vi "WriteAndClosePatientDateInfoFile.vi"(8 "error in (no error)":errorcluster, 10 "date_specific_info":T1, 11 "file path (use dialog)":path) -> (0 "error out":errorcluster)   [LabVIEW 2013, in "main.lvlib"]
uses:
  main.lvlib
  Controls/date_specific_info.ctl
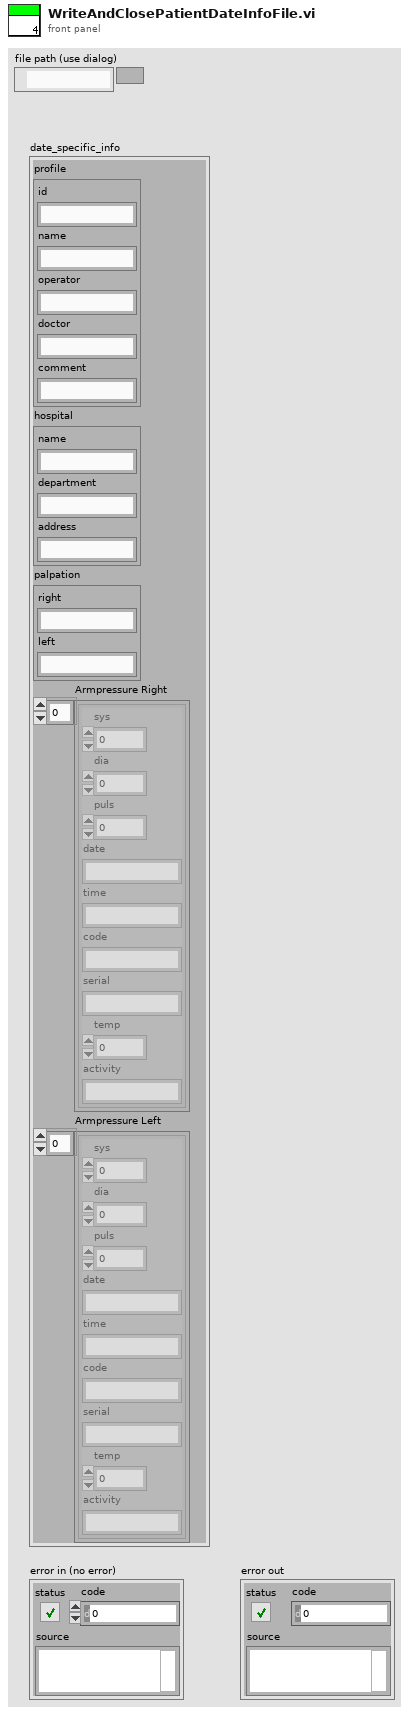
[diagram p1: front panel]
types:
  T1 = typedef "main.lvlib/date_specific_info.ctl" = cluster{"profile":cluster{"id":string, "name":string, "operator":string, "doctor":string, "comment":string}, "hospital":cluster{"name":string, "department":string, "address":string}, "palpation":cluster{"right":string, "left":string}, "Armpressure Right":cluster{"sys":dbl, "dia":dbl, "puls":dbl, "date":string, "time":string, "code":string, "serial":string, "temp":dbl, "activity":string}[], "Armpressure Left":cluster{"sys":dbl, "dia":dbl, "puls":dbl, "date":string, "time":string, "code":string, "serial":string, "temp":dbl, "activity":string}[]}
  T2 = enum16{"open", "replace", "create", "open or create", "replace or create", "replace or create with confirmation"}
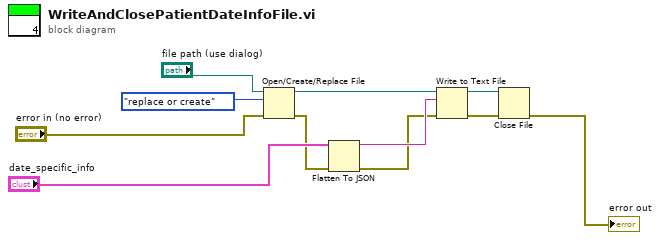
[diagram p0: block diagram]
diagram:
  n1 = Open/Create/Replace File(file path (use dialog)="file path (use dialog)", error in="error in (no error)", operation (0:open)=T2."replace or create") -> (refnum out=w3:refnum<file>, error out=w2:errorcluster)  [unwired: 3 in, 1 out]
  n2 = Flatten To JSON(anything="date_specific_info", error in (no error)=w2) -> (JSON string=w8:string, 11:w1:errorcluster)  [unwired: 1 in]
  n3 = Write to Text File(file (use dialog)=w3, text=w8, error in=w1) -> (refnum out=w9:refnum<file>, error out=w10:errorcluster)  [unwired: 1 in, 1 out]
  n4 = Close File(refnum=w9, error in=w10) -> (error out=→"error out":errorcluster)  [unwired: 1 out]
